vi "BPM Calculator.vi"(11 "waveform in":waveform(dbl)) -> (3 "Numeric":dbl)   [LabVIEW 2023]
uses:
  <vilib>/measure/matone.llb/Extract Single Tone Information 1 Chan.vi
  <vilib>/measure/NI_MAPro.lvlib
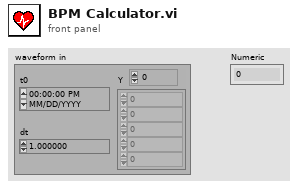
[diagram p1: front panel]
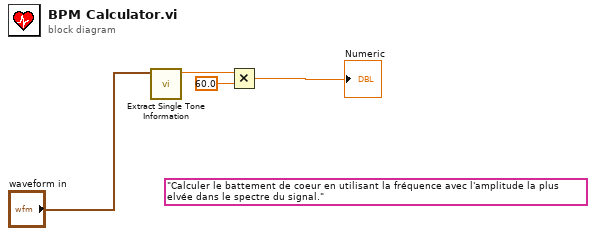
[diagram p0: block diagram]
diagram:
  (unwired) "Calculer le battement de coeur en utilisant la fréquence avec l'amplitude la plus elvée dans le spectre du signal."
  n1 = call-poly <vilib>:"Extract Single Tone Information.vi"("time signal in"="waveform in") -> ("detected frequency"=w2:dbl)  [unwired: 5 in, 5 out]
  n2 = Multiply(x=w2, y=60.0) -> (x*y=→"Numeric":dbl)
